vi "AMC QR Get All Queues.vi"(8 "error in (no error)":errorcluster) -> (0 "error out":errorcluster, 1 "Number of Queues":i32, 2 "All Properties":T1[](array[typedef]), 3 "All Queues":T2[](array[typedef]))   [LabVIEW 2015]
doc: "This VI is used for compatibility with previous versions of the AMC library. Use the AMC VIs located in the <b>Data Communication >> Asynchronous Message Communication</b> palette."
uses:
  <vilib>/NI/AMC/Message Queue.ctl
  <vilib>/NI/AMC/Message.ctl
  <vilib>/NI/Tools/Keyed Array/KeyedArray.ctl
  <vilib>/NI/AMC/Queue Registry Properties.ctl
  <vilib>/Utility/error.llb/Clear Errors.vi
  <vilib>/NI/AMC/Queue Registry.vi
  <vilib>/NI/AMC/AMC.lvlib
  <vilib>/NI/Tools/Keyed Array/Tools_KeyedArray.lvlib
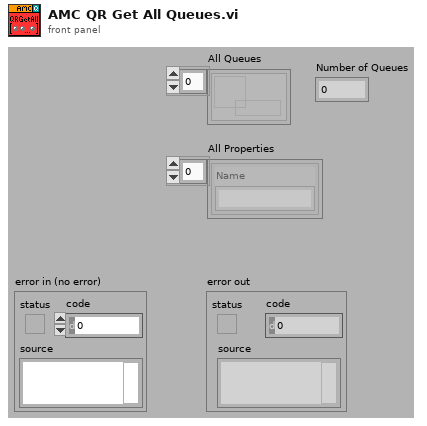
[diagram p1: front panel]
types:
  T1 = typedef "AMC.lvlib/Queue Registry Properties.ctl" = cluster{"Name":string}
  T2 = typedef "AMC.lvlib/Message Queue.ctl" = refnum<queue>
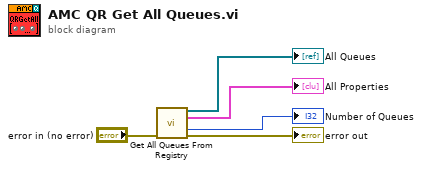
[diagram p0: block diagram]
diagram:
  n1 = call <vilib>:"Get All Queues From Registry.vi"("error in"="error in (no error)") -> ("all queues"=→"All Queues":T2[], "all properties"=→"All Properties":T1[], "number of queues"=→"Number of Queues":i32, "error out"=→"error out":errorcluster)  [unwired: 11 in]
